vi "DumbDash Save Values.vi"(9 "Message Box":refnum<vi>, 11 "Controls In":T1[](array[typedef])) -> ()   [LabVIEW 2014]
uses:
  DumbDash Control.ctl
  DumbDash Control Type.ctl
  <vilib>/Utility/sysdir.llb/System Directory Type.ctl
  <vilib>/Utility/config.llb/Write Key (Double).vi
  <vilib>/Utility/config.llb/Write Key (Boolean).vi
  <vilib>/Utility/config.llb/Write Key (String).vi
  <vilib>/Utility/config.llb/NI_LVConfig.lvlib
panel:
  out "file created?":bool
  out "file path":path
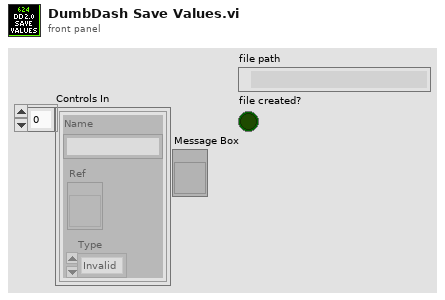
[diagram p1: front panel]
types:
  T1 = typedef "DumbDash Control.ctl" = cluster{"Name":string, "Ref":refnum<vi>, "Type":T2}
  T2 = typedef "DumbDash Control Type.ctl" = enum16{"Invalid", "Number", "Boolean", "String"}
  T3 = typedef "System Directory Type.ctl" = i32
  T4 = typedef "NI_LVConfig.lvlib/Config Data RefNum.ctl" = refnum<k1>
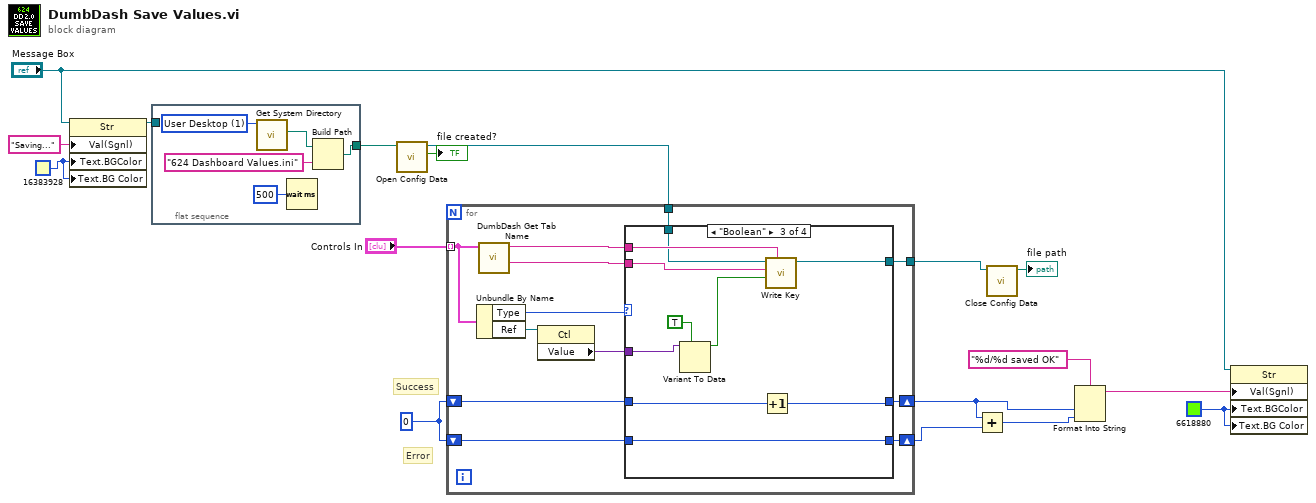
[diagram p0: block diagram]
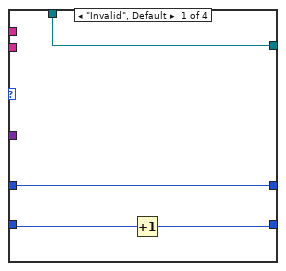
[diagram p2: hidden frame]
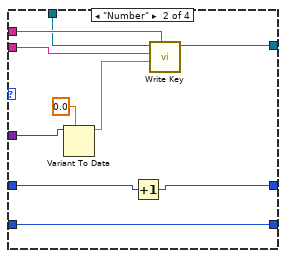
[diagram p3: hidden frame]
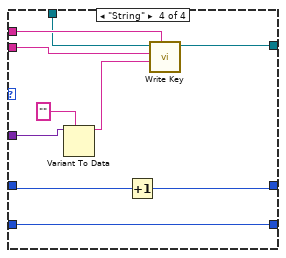
[diagram p4: hidden frame]
diagram:
  w2 = u32 16383928
  w5 = u32 6618880
  w11 = 0
  # "Error"
  # "Success"
  n1 = property class="Str"(reference="Message Box", "Val(Sgnl)"="Saving..." ("Text.Text"), "Text.BGColor"=w2, "Text.BG Color"=w2) -> (reference out=w1:refnum<vi>)  [unwired: 1 in, 1 out]
  n2 = flat-sequence {
    tunnel: [w19] -> w12
    tunnel: w1 -> [_]
    frame #0 {
      w22 = T3 1 items=["User Home"=0, "User Desktop"=1, "User Documents"=2, "User Application Data"=3, "User Preferences"=4, "User Temporary"=5, "Public Documents"=6, "Public Application Data"=7, "Public Preferences"=8, "Public Cache"=13, "System Core Libraries"=9, "System Installed Libraries"=10, "Application Files"=11, "Boot Volume Root"=12] ("system directory type")
      n3 = call <vilib>:"Get System Directory.vi"("system directory type"=w22) -> ("system directory"=w21:path)  [unwired: 10 in]
      n4 = Wait (ms)(milliseconds to wait=u32 500) -> ()  [unwired: 1 out]
      n5 = Build Path(base path=w21, name or relative path="624 Dashboard Values.ini") -> (appended path=w19:path)
    }
  }
  n6 = call <vilib>:"Open Config Data.vi"("configuration file path"=w12) -> ("file created?"=→"file created?":bool, "refnum"=w16:T4)  [unwired: 8 in, 1 out]
  n7 = for {
    tunnel: "Controls In" -> [w30] mode=indexing
    tunnel: w16 -> [w33]
    tunnel: [w27] -> w15
    shift-right: [w23] -> w9
    shift-left: w11 -> [w24]
    shift-right: [w25] -> w8
    shift-left: w11 -> [w26]
    n8 = Unbundle By Name(w30) -> ("Type"=w31:T2, "Ref"=w29:refnum<vi>)
    n9 = call "DumbDash Get Tab Name.vi"("Cluster"=w30) -> ("Rest of Name"=w32:string, "Tab Name"=w34:string)  [unwired: 9 in]
    n10 = property class="Ctl"(reference=w29) -> ("Value"=w28:variant)  [unwired: 1 in, 2 out]
    n11 = case shown="\"Boolean\"" w31 {
      tunnel: w34 -> [_ w48 w58 w68]
      tunnel: w33 -> [w38 w47 w57 w67]
      tunnel: w32 -> [_ w46 w56 w66]
      tunnel: w28 -> [_ w45 w55 w65]
      tunnel: [w38 w42 w52 w62] -> w27
      tunnel: w26 -> [w35 w40 w51 w61]
      tunnel: [w35 w39 w50 w60] -> w25
      tunnel: w24 -> [w37 w41 w49 w59]
      tunnel: [w36 w41 w49 w59] -> w23
      frame "Invalid", Default {
        n12 = Increment(x=w37) -> (x+1=w36:i32)
      }
      frame "Number" {
        n13 = Variant To Data(type=0.0, Variant=w45) -> (data=w43:dbl)  [unwired: 1 in, 1 out]
        n14 = Increment(x=w40) -> (x+1=w39:i32)
        n15 = call-poly <vilib>:"Write Key.vi"("section"=w48, "value"=w43, "key"=w46, "refnum"=w47) -> ("refnum out"=w42:T4)  [unwired: 5 in, 2 out]
      }
      frame "Boolean" {
        n16 = Variant To Data(type=TRUE, Variant=w55) -> (data=w54:bool)  [unwired: 1 in, 1 out]
        n17 = Increment(x=w51) -> (x+1=w50:i32)
        n18 = call-poly <vilib>:"Write Key.vi"("section"=w58, "value"=w54, "key"=w56, "refnum"=w57) -> ("refnum out"=w52:T4)  [unwired: 5 in, 2 out]
      }
      frame "String" {
        n19 = Variant To Data(type="", Variant=w65) -> (data=w64:string)  [unwired: 1 in, 1 out]
        n20 = Increment(x=w61) -> (x+1=w60:i32)
        n21 = call-poly <vilib>:"Write Key.vi"("section"=w68, "value"=w64, "key"=w66, "refnum"=w67) -> ("refnum out"=w62:T4)  [unwired: 5 in, 2 out]
      }
    }
  }
  n22 = Add(x=w8, y=w9) -> (x+y=w7:i32)
  n23 = call <vilib>:"Close Config Data.vi"("refnum"=w15) -> ("file path"=→"file path":path)  [unwired: 9 in, 1 out]
  n24 = Format Into String(format string="%d/%d saved OK", w8, w7) -> (resulting string=w6:string)  [unwired: 2 in, 1 out]
  n25 = property class="Str"(reference="Message Box", "Val(Sgnl)"=w6, "Text.BGColor"=w5, "Text.BG Color"=w5) -> ()  [unwired: 1 in, 2 out]
